vi "Example Callback - Quaternion Callback.vi"(4 "Quaternion":refnum<user-event>, 5 "Event Data":T1, 6 "Control Ref":refnum<k24>, 7 "Event Common Data":T2) -> ()   [LabVIEW 2013]
uses:
  C:/tf/play/labview/Tinkerforge.dll
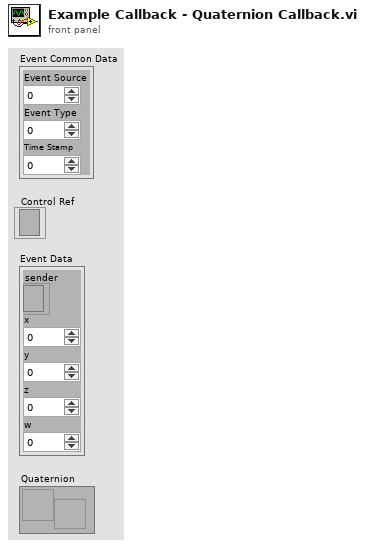
[diagram p1: front panel]
types:
  T1 = cluster{"sender":refnum<k24>, "x":sgl, "y":sgl, "z":sgl, "w":sgl}
  T2 = cluster{"Event Source":i32, "Event Type":u32, "Time Stamp":u32}
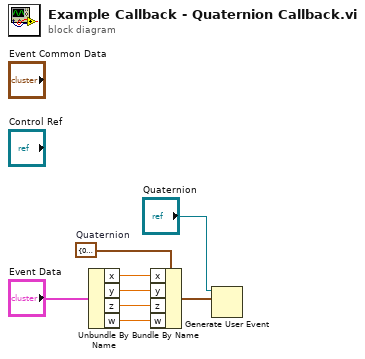
[diagram p0: block diagram]
diagram:
  w7 = cluster{"x":sgl, "y":sgl, "z":sgl, "w":sgl} {"x"=0.0, "y"=0.0, "z"=0.0, "w"=0.0}  # Quaternion
  n1 = Unbundle By Name("Event Data") -> ("x"=w5:sgl, "y"=w4:sgl, "z"=w3:sgl, "w"=w2:sgl)
  n2 = Bundle By Name(cluster=w7, "x"=w5, "y"=w4, "z"=w3, "w"=w2) -> (w6:cluster{"x":sgl, "y":sgl, "z":sgl, "w":sgl})
  n3 = Generate User Event(user event="Quaternion", event data cluster=w6) -> ()  [unwired: 2 in, 2 out]
